vi "IOApi.vi"(9 "GameCommand From Hardware":T1, 11 "Playfield From Software":bool[][](array[boolean])) -> (1 "GameCommand To Software":T1, 3 "Playfield To Hardware":bool[][](array[boolean]))   [LabVIEW 2026]
doc: "This VI functions as an API for connecting the hardware the software part of the application."
uses:
  01_Typen/GameCommandTypeDef.ctl
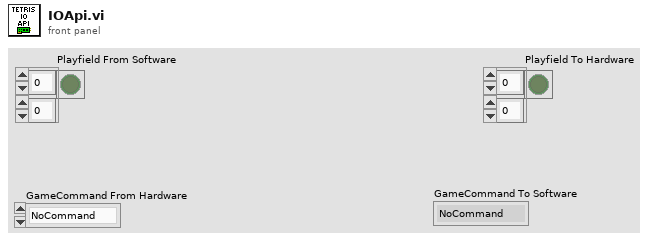
[diagram p1: front panel]
types:
  T1 = typedef "GameCommandTypeDef.ctl" = enum16{"NoCommand", "Rotate", "MoveLeft", "MoveRight"}
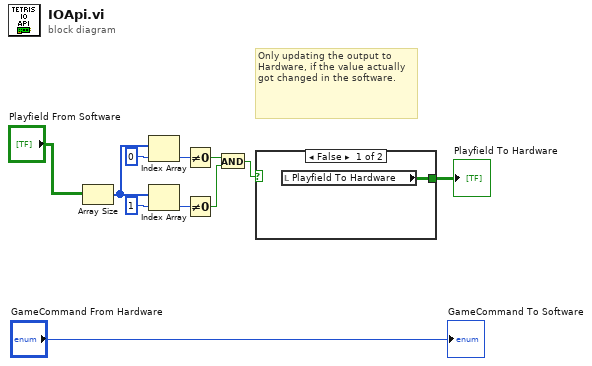
[diagram p0: block diagram]
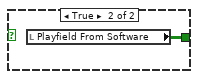
[diagram p2: hidden frame]
diagram:
  # "Only updating the output to Hardware, if the value actually got changed in the software."
  n1 = Array Size(array="Playfield From Software") -> (size(s)=w9:i32[])
  n2 = Index Array(array=w9, index=0) -> (element=w5:i32)
  n3 = Index Array(array=w9, index=1) -> (element=w6:i32)
  n4 = Not Equal To 0?(x=w5) -> (x != 0?=w3:bool)
  n5 = Not Equal To 0?(x=w6) -> (x != 0?=w4:bool)
  n6 = And(x=w3, y=w4) -> (x .and. y?=w2:bool)
  n7 = case shown="False" w2 {
    tunnel: [w12 w13] -> w1
    frame False {
      n8 = local read "Playfield To Hardware"() -> (w12:bool[][])
    }
    frame True {
      n9 = local read "Playfield From Software"() -> (w13:bool[][])
    }
  }
  "Playfield To Hardware" <- w1
  "GameCommand To Software" <- "GameCommand From Hardware"
